vi "Periodic Tasks.vi"   [LabVIEW 2014]
doc: "This VI runs in parallel to other tasks. It can contain as many user-defined periodic loops as you need. These can carry out PID or other sorts of timed response."
uses:
  Robot Global Data.vi
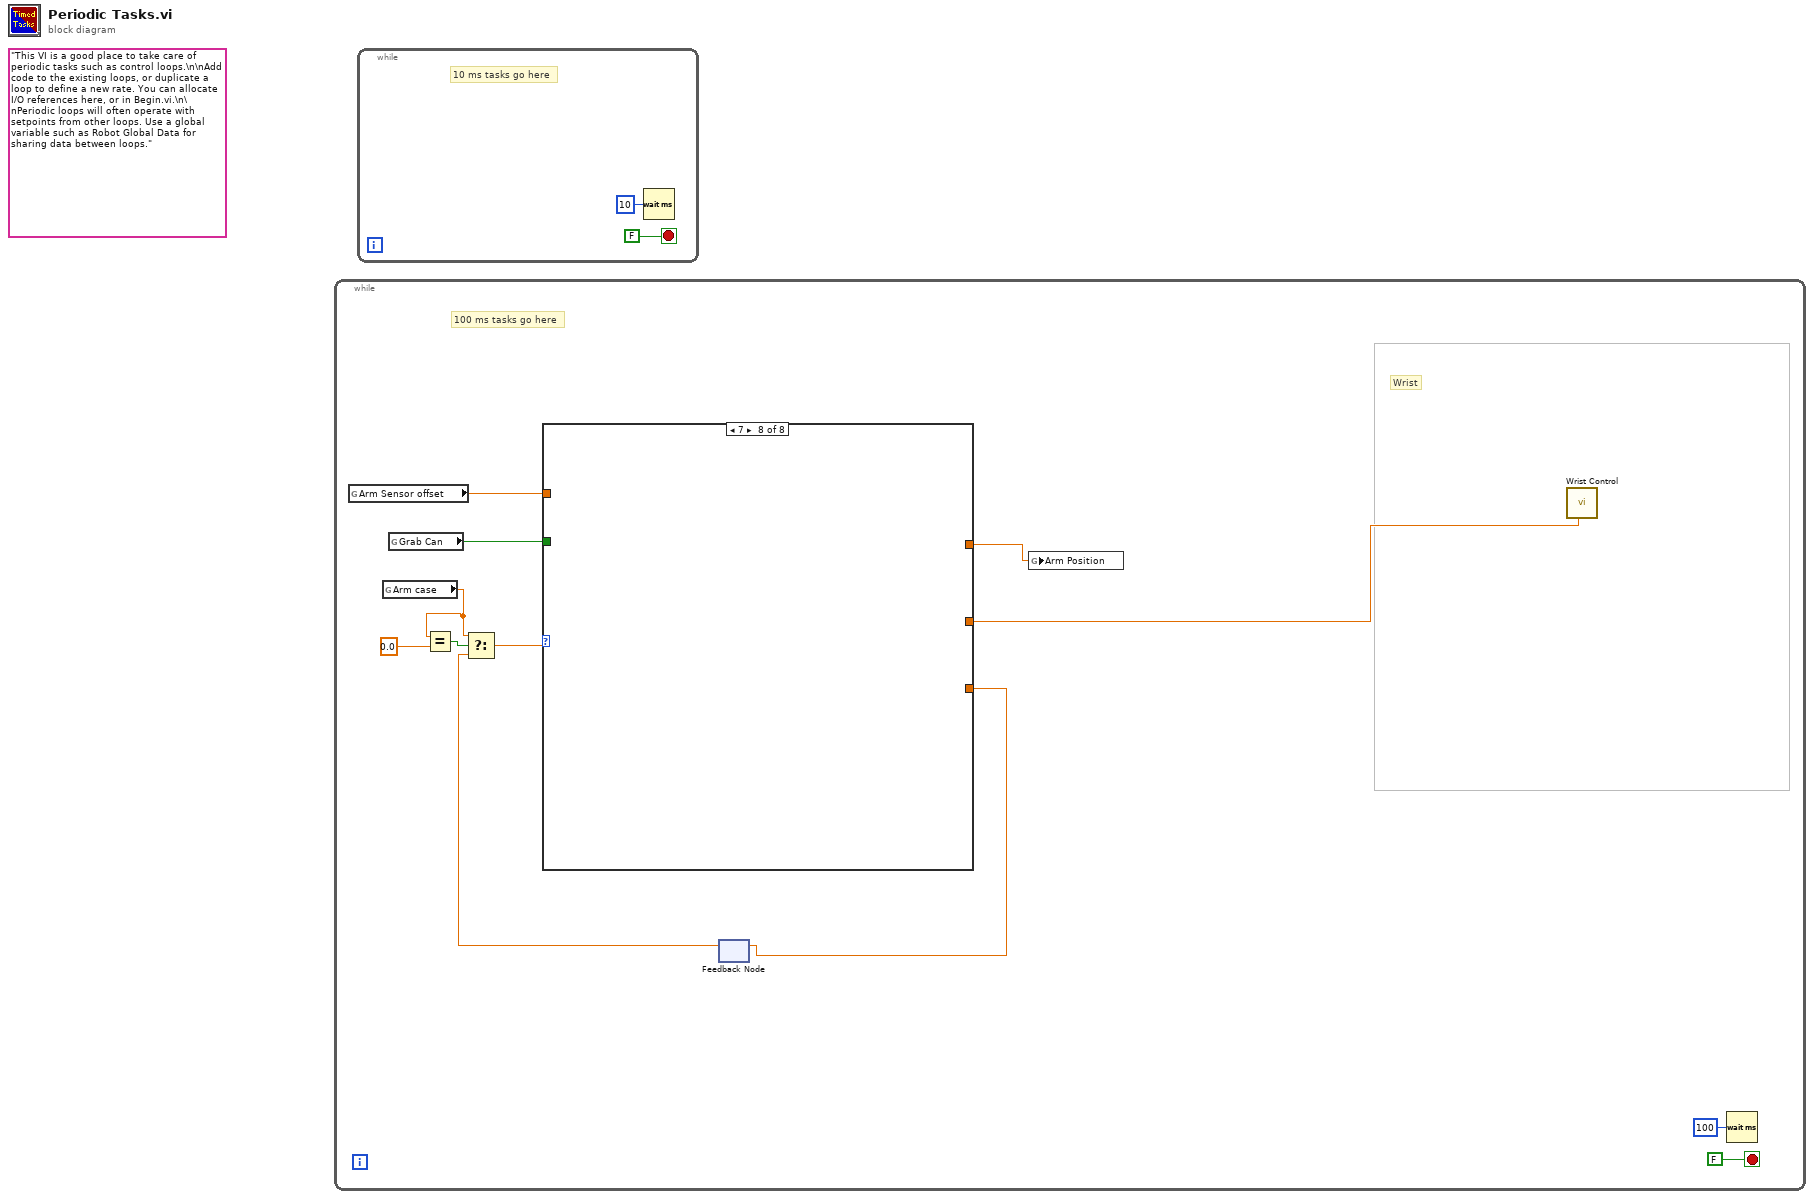
[diagram p0: block diagram]
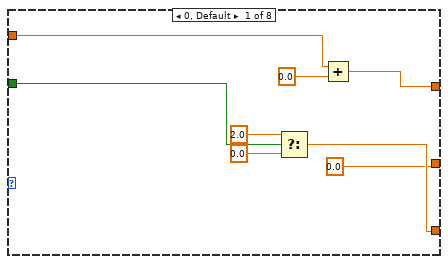
[diagram p2: hidden frame]
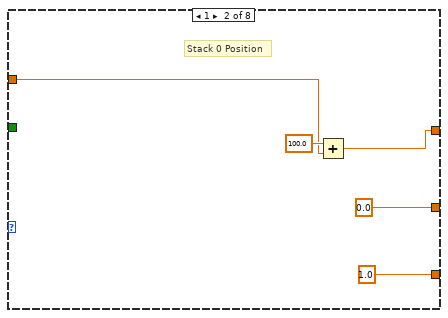
[diagram p3: hidden frame]
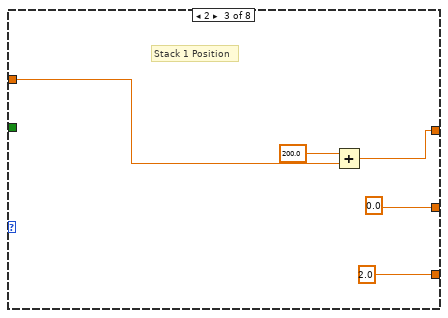
[diagram p4: hidden frame]
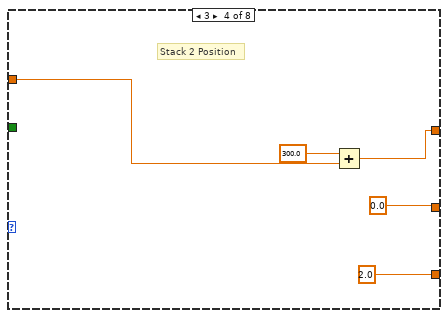
[diagram p5: hidden frame]
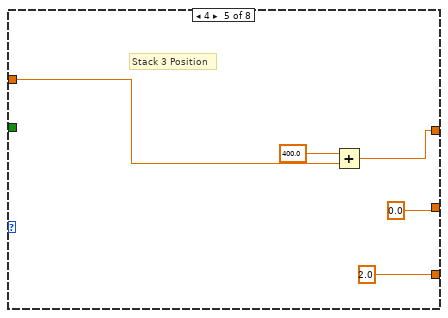
[diagram p6: hidden frame]
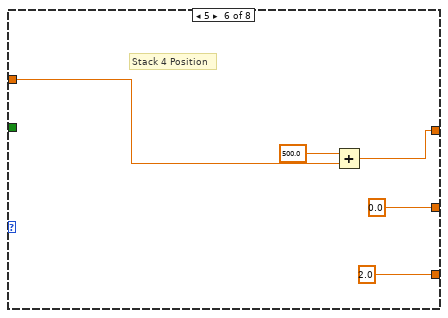
[diagram p7: hidden frame]
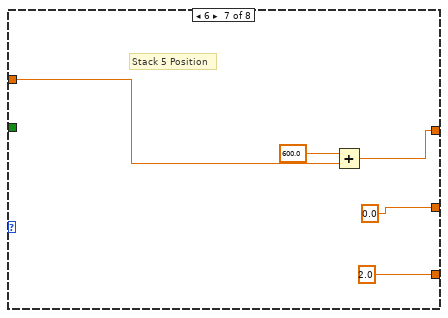
[diagram p8: hidden frame]
diagram:
  (unwired) "This VI is a good place to take care of periodic tasks such as control loops.\n\nAdd code to the existing loops, or duplicate a loop to define a new rate. You can allocate I/O references here, or in Begin.vi.\n\nPeriodic loops will often operate with setpoints from other loops. Use a global variable such as Robot Global Data for sharing data between loops."
  n1 = while {
    stop <- FALSE stop-if-true
    # "Wrist"
    # "100 ms tasks go here"
    n2 = global read "Robot Global Data.vi" "Arm Sensor offset"() -> (w3:dbl)
    n3 = global read "Robot Global Data.vi" "Arm case"() -> (w7:dbl)
    n4 = global read "Robot Global Data.vi" "Grab Can"() -> (w1:bool)
    n5 = Equal?(x=w7, y=0.0) -> (x = y?=w9:bool)
    n6 = feedback #1() -> (w5:dbl)  [unwired: 1 in]
    n7 = Select(t=w7, s=w9, f=w5) -> (s? t:f=w8:dbl)
    n8 = case shown="7" w8 {
      tunnel: [w14 1.0 2.0 2.0 2.0 2.0 2.0 _] -> w6
      tunnel: [w19 w22 w27 w32 w37 w42 w47 _] -> w4
      tunnel: w3 -> [w20 w23 w29 w34 w39 w44 w49 _]
      tunnel: [0.0 0.0 0.0 0.0 0.0 0.0 0.0 _] -> w2
      tunnel: w1 -> [w17 _ _ _ _ _ _ _]
      frame 0, Default {
        n9 = Select(t=2.0, s=w17, f=0.0) -> (s? t:f=w14:dbl)
        n10 = Add(x=w20, y=0.0) -> (x+y=w19:dbl)
      }
      frame 1 {
        # "Stack 0 Position"
        n11 = Add(x=100.0, y=w23) -> (x+y=w22:dbl)
      }
      frame 2 {
        # "Stack 1 Position"
        n12 = Add(x=200.0, y=w29) -> (x+y=w27:dbl)
      }
      frame 3 {
        # "Stack 2 Position"
        n13 = Add(x=300.0, y=w34) -> (x+y=w32:dbl)
      }
      frame 4 {
        # "Stack 3 Position"
        n14 = Add(x=400.0, y=w39) -> (x+y=w37:dbl)
      }
      frame 5 {
        # "Stack 4 Position"
        n15 = Add(x=500.0, y=w44) -> (x+y=w42:dbl)
      }
      frame 6 {
        # "Stack 5 Position"
        n16 = Add(x=600.0, y=w49) -> (x+y=w47:dbl)
      }
      frame 7 {
      }
    }
    n17 = feedback-in #1(w6) -> ()
    n18 = global write "Robot Global Data.vi" "Arm Position"(w4) -> ()
    n19 = call "Wrist Control.vi"("Case for Wrist"=w2) -> ()  [unwired: 9 in, 2 out]
    n20 = Wait (ms)(milliseconds to wait=u32 100) -> ()  [unwired: 1 out]
  }
  n21 = while {
    stop <- FALSE stop-if-true
    # "10 ms tasks go here"
    n22 = Wait (ms)(milliseconds to wait=u32 10) -> ()  [unwired: 1 out]
  }
